vi "CUBED_JOYSTICK.vi"(11 "axis input":dbl) -> (3 "axis output":dbl)   [LabVIEW 2014]
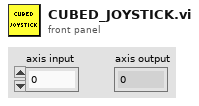
[diagram p1: front panel]
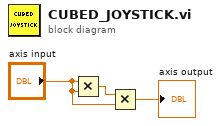
[diagram p0: block diagram]
diagram:
  n1 = Multiply(x="axis input", y="axis input") -> (x*y=w1:dbl)
  n2 = Multiply(x=w1, y="axis input") -> (x*y=→"axis output":dbl)
